vi "Drive Initialize.vi"(11 "Motor CAN IDs":T15={"Left Leader"=1, "Left Follower 1"=2, "Left Follower 2"=3, "Right Leader"=4, "Right Follower 1"=3, "Right Follower 2"=4}) -> (0 "Right Motor":T1={"DeviceStatus"={"status"=FALSE, "code"=0, "source"=""}, "Type"=enum."PWM", "PWM"={"PWM Channel"=enum."Invalid", "DeadBand"={"Name"="", "maxPositivePwm"=0, "minPositivePwm"=0, "centerPwm"=0, "maxNegativePwm"=0, "minNegativePwm"=0, "angularRange"=0}}, "CAN"={"Device Number"=0, "SetOutput VI Ref"=variant(refnum<vi> refnum), "GetOutput VI Ref"=variant(refnum<vi> refnum), "Enable VI Ref"=variant(refnum<vi> refnum), "Disable VI Ref"=variant(refnum<vi> refnum), "Data"=variant}, "Invert"=FALSE, "DIO PWM"={"PWM \"Enable\" Channel"=enum."Invalid", "DIOChannel"=enum."Invalid", "PWM Rate"=0.0}}, 1 "Left Motor":T1={"DeviceStatus"={"status"=FALSE, "code"=0, "source"=""}, "Type"=enum."PWM", "PWM"={"PWM Channel"=enum."Invalid", "DeadBand"={"Name"="", "maxPositivePwm"=0, "minPositivePwm"=0, "centerPwm"=0, "maxNegativePwm"=0, "minNegativePwm"=0, "angularRange"=0}}, "CAN"={"Device Number"=0, "SetOutput VI Ref"=variant(refnum<vi> refnum), "GetOutput VI Ref"=variant(refnum<vi> refnum), "Enable VI Ref"=variant(refnum<vi> refnum), "Disable VI Ref"=variant(refnum<vi> refnum), "Data"=variant}, "Invert"=FALSE, "DIO PWM"={"PWM \"Enable\" Channel"=enum."Invalid", "DIOChannel"=enum."Invalid", "PWM Rate"=0.0}}, 2 "imu":T6={"DevStatus"={"status"=FALSE, "code"=0, "source"=""}, "Hardware Config"={"SPI Clock Rate (Hz)"=1000000.0, "IMU SPI Mode (3)"=enum."Mode 3 (Clk Idle High,Sample on Trailing)", "IMU Reset Pin"=enum."SPI Port CS2", "IMU SPI Bus"=enum."SPI On-Board, CS0", "IMU Data Ready Pin"=enum."SPI Port CS1", "Stall Config"={"Pow2BytesPerRead"=255, "StallTicks"=640, "CsToSclkTicks"=5}, "IMU Status LED Pin"=enum."DIO MXP 9"}, "Calibration Complete"=refnum, "Status FIFO"=refnum, "Last Value Reference"=refnum, "Sychronous Process VI"=refnum, "Cmd FIFO"=refnum, "Source"={"DevStatus"={"status"=FALSE, "code"=0, "source"=""}, "AnalogTriggerMode?"=FALSE, "DigitalMode"={"DIO Channel"=enum."Disabled"}, "AnalogTriggerMode"={"AnalogTriggerIndex"=enum."Trig 0", "OutputType"=enum."InWindow"}}, "Data FIFO"=refnum, "IMU Status LED Pin"=enum."DIO MXP 9", "Calibration Time"=0}, 3 "Drive":T16)   [LabVIEW 2019]
uses:
  <vilib>/Rock Robotics/WPI/RobotDrive/WPI_RobotDriveDevRef.ctl
  <vilib>/Rock Robotics/WPI/MotorControl/WPI_MotorControlDeviceRef.ctl
  <vilib>/Rock Robotics/WPI/MotorControl/WPI_MotorControlType.ctl
  <vilib>/Rock Robotics/SystemInterfaces/DIO/FPGA_DIOPWMChannel.ctl
  <vilib>/Rock Robotics/WPI/PWM/WPI_PWMDeadband.ctl
  <vilib>/Rock Robotics/SystemInterfaces/DIO/FPGA_DIOChannel.ctl
  <vilib>/Rock Robotics/WPI/ThirdParty/ADI/ADIS16448/Typedef/ADIS16448 Device Reference.ctl
  <vilib>/Rock Robotics/WPI/ThirdParty/ADI/ADIS16448/Typedef/ADIS16448 Hardware Configuration.ctl
  <vilib>/Rock Robotics/WPI/SPI/WPI_SPIMode.ctl
  <vilib>/Rock Robotics/SystemInterfaces/spilib/spi_bus.ctl
  <vilib>/Rock Robotics/WPI/ThirdParty/ADI/ADIS16448/Typedef/ADIS16448 Status.ctl
  <vilib>/Rock Robotics/WPI/ThirdParty/ADI/ADIS16448/Typedef/ADIS16448 Data.ctl
  <vilib>/Rock Robotics/WPI/ThirdParty/ADI/ADIS16448/Typedef/ADIS16448 Process.ctl
  <vilib>/Rock Robotics/WPI/ThirdParty/ADI/ADIS16448/Typedef/ADIS16448 Command Type.ctl
  <vilib>/Rock Robotics/SystemInterfaces/CounterEncoderSourceConvertion/FPGA_CounterEncoderSourceConvertionLVSourceType.ctl
  <vilib>/Rock Robotics/SystemInterfaces/DIO/FPGA_DIODigitalSourceChannel.ctl
  <vilib>/Rock Robotics/SystemInterfaces/AnalogTrigger/FPGA_AnalogTriggerIndex.ctl
  <vilib>/Rock Robotics/SystemInterfaces/AnalogTrigger/FPGA_AnalogTriggerOutType.ctl
  <vilib>/Rock Robotics/WPI/SafetyOutput/WPI_SafetyOutputConfigMenu.ctl
  <vilib>/Rock Robotics/WPI/ThirdParty/REV Robotics/SPARK MAX/Typedef/Spark MAX Motor Type.ctl
  <vilib>/Rock Robotics/WPI/RobotDrive/WPI_RobotDriveOpen2MotorWithExistingMotors.vi
  Drive Published Globals.vi
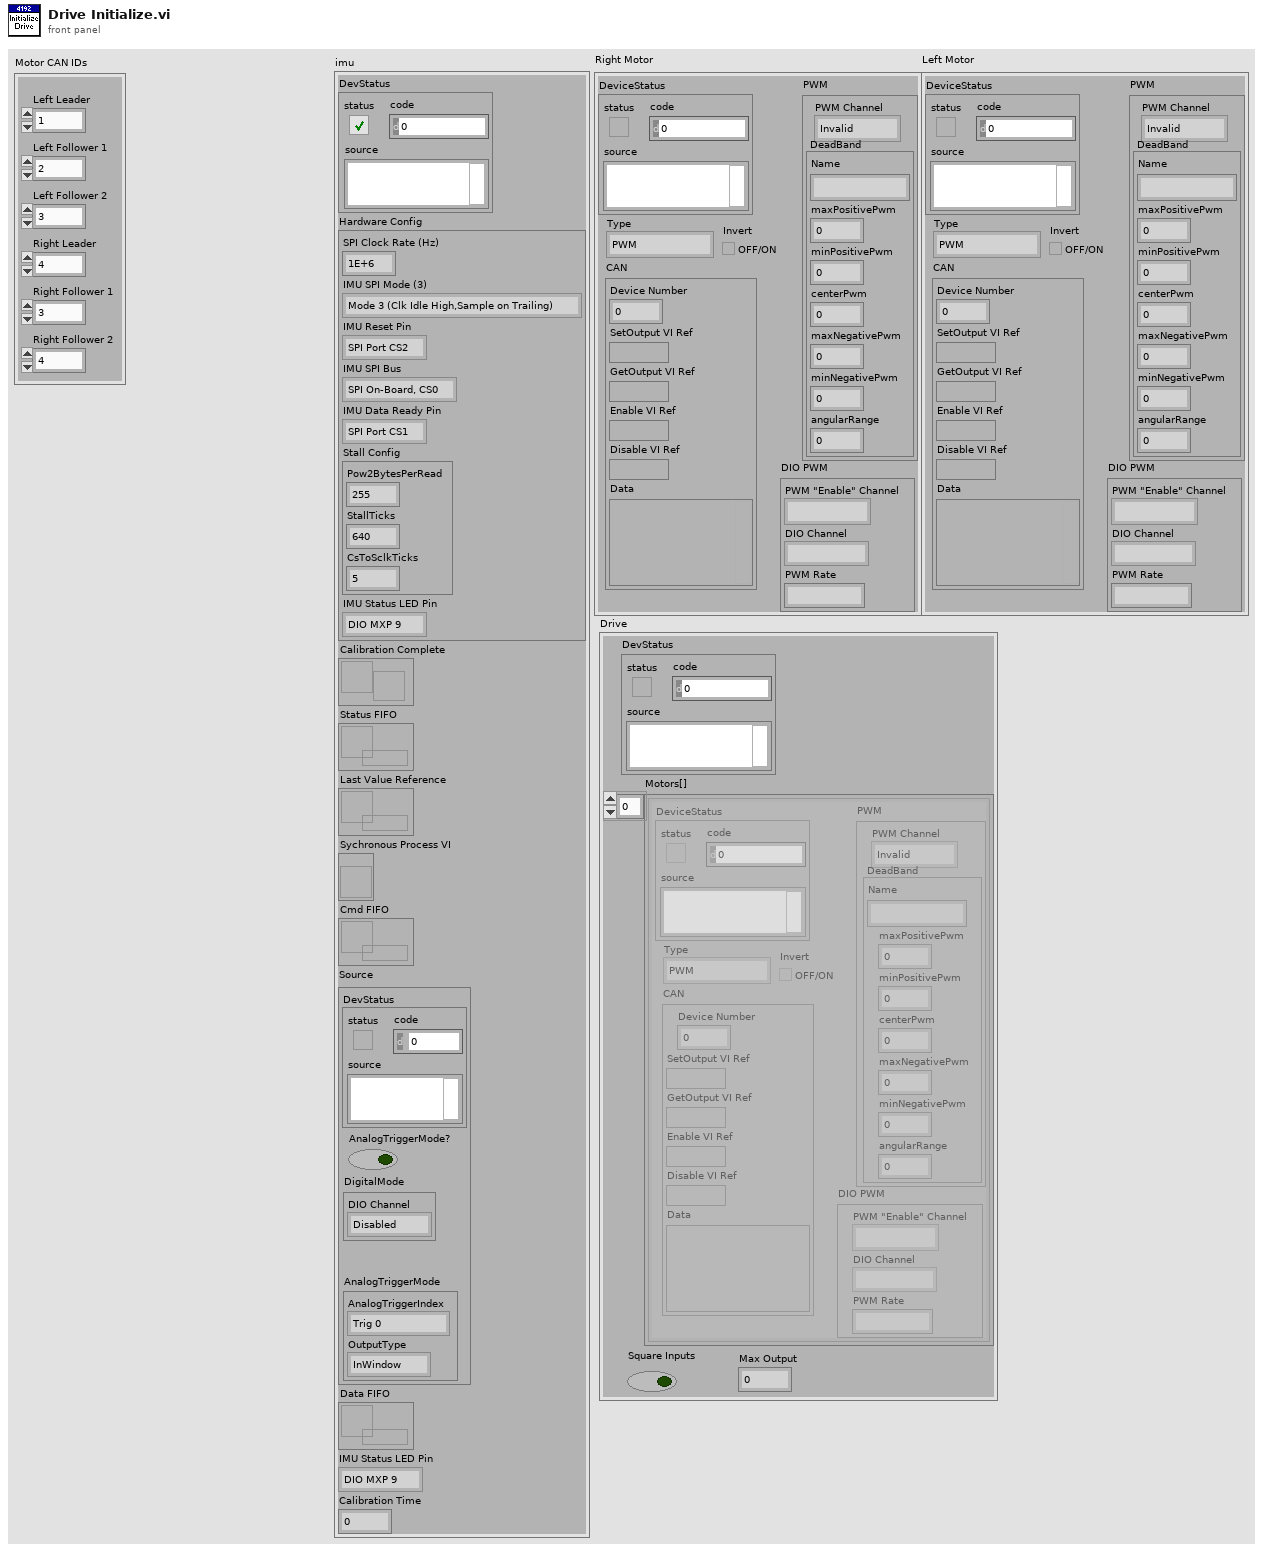
[diagram p1: front panel]
types:
  T1 = typedef "WPI_MotorControlDeviceRef.ctl" = cluster{"DeviceStatus":errorcluster, "Type":T2, "PWM":cluster{"PWM Channel":T3, "DeadBand":T4}, "CAN":cluster{"Device Number":u8, "SetOutput VI Ref":variant, "GetOutput VI Ref":variant, "Enable VI Ref":variant, "Disable VI Ref":variant, "Data":variant}, "Invert":bool, "DIO PWM":cluster{"PWM \"Enable\" Channel":T3, "DIOChannel":T5, "PWM Rate":dbl}}
  T2 = typedef "WPI_MotorControlType.ctl" = enum16{"PWM", "CAN", "DIO PWM"}
  T3 = typedef "FPGA_DIOPWMChannel.ctl" = enum8{"PWM 0", "PWM 1", "PWM 2", "PWM 3", "PWM 4", "PWM 5", "PWM 6", "PWM 7", "PWM 8", "PWM 9", "PWM MXP 0", "PWM MXP 1", "PWM MXP 2", "PWM MXP 3", "PWM MXP 4", "PWM MXP 5", "PWM MXP 6", "PWM MXP 7", "PWM MXP 8", "PWM MXP 9", "Invalid"}
  T4 = typedef "WPI_PWMDeadband.ctl" = cluster{"Name":string, "maxPositivePwm":i32, "minPositivePwm":i32, "centerPwm":i32, "maxNegativePwm":i32, "minNegativePwm":i32, "angularRange":u16}
  T5 = typedef "FPGA_DIOChannel.ctl" = enum8{"DIO 0", "DIO 1", "DIO 2", "DIO 3", "DIO 4", "DIO 5", "DIO 6", "DIO 7", "DIO 8", "DIO 9", "DIO MXP 0", "DIO MXP 1", "DIO MXP 2", "DIO MXP 3", "DIO MXP 4", "DIO MXP 5", "DIO MXP 6", "DIO MXP 7", "DIO MXP 8", "DIO MXP 9", "DIO MXP 10", "DIO MXP 11", "DIO MXP 12", "DIO MXP 13", "DIO MXP 14", "DIO MXP 15", "SPI Port CS1", "SPI Port CS2", "SPI Port CS3", "SPI Port MISO", "SPI Port MOSI", "Invalid"}
  T6 = typedef "ADIS16448 Device Reference.ctl" = cluster{"DevStatus":errorcluster, "Hardware Config":T7, "Calibration Complete":refnum<notifier>, "Status FIFO":refnum<k33>, "Last Value Reference":refnum<data-value>, "Sychronous Process VI":T10, "Cmd FIFO":refnum<k33>, "Source":T11, "Data FIFO":refnum<k33>, "IMU Status LED Pin":T5, "Calibration Time":u32}
  T7 = typedef "ADIS16448 Hardware Configuration.ctl" = cluster{"SPI Clock Rate (Hz)":dbl, "IMU SPI Mode (3)":T8, "IMU Reset Pin":T5, "IMU SPI Bus":T9, "IMU Data Ready Pin":T5, "Stall Config":cluster{"Pow2BytesPerRead":u8, "StallTicks":u16, "CsToSclkTicks":u8}, "IMU Status LED Pin":T5}
  T8 = typedef "WPI_SPIMode.ctl" = enum16{"Mode 0 (Clk Idle Low,Sample on Leading)", "Mode 1 (Clk Idle Low,Sample on Trailing)", "Mode 2 (Clk Idle High,Sample on Leading)", "Mode 3 (Clk Idle High,Sample on Trailing)"}
  T9 = typedef "spi_bus.ctl" = enum16{"SPI On-Board, CS0", "SPI On-Board, CS1", "SPI On-Board, CS2", "SPI On-Board, CS3", "SPI MXP", "Invalid"}
  T10 = typedef "ADIS16448 Process.ctl" = refnum<vi>
  T11 = typedef "FPGA_CounterEncoderSourceConvertionLVSourceType.ctl" = cluster{"DevStatus":errorcluster, "AnalogTriggerMode?":bool, "DigitalMode":cluster{"DIO Channel":T12}, "AnalogTriggerMode":cluster{"AnalogTriggerIndex":T13, "OutputType":T14}}
  T12 = typedef "FPGA_DIODigitalSourceChannel.ctl" = enum8{"DIO 0", "DIO 1", "DIO 2", "DIO 3", "DIO 4", "DIO 5", "DIO 6", "DIO 7", "DIO 8", "DIO 9", "DIO MXP 0", "DIO MXP 1", "DIO MXP 2", "DIO MXP 3", "DIO MXP 4", "DIO MXP 5", "DIO MXP 6", "DIO MXP 7", "DIO MXP 8", "DIO MXP 9", "DIO MXP 10", "DIO MXP 11", "DIO MXP 12", "DIO MXP 13", "DIO MXP 14", "DIO MXP 15", "SPI Port CS1", "SPI Port CS2", "SPI Port CS3", "SPI Port MISO", "SPI Port MOSI", "Disabled"}
  T13 = typedef "FPGA_AnalogTriggerIndex.ctl" = enum8{"Trig 0", "Trig 1", "Trig 2", "Trig 3", "Trig 4", "Trig 5", "Trig 6", "Trig 7", "Invalid"}
  T14 = typedef "FPGA_AnalogTriggerOutType.ctl" = enum16{"InWindow", "TriggerState", "Rising", "Falling"}
  T15 = cluster{"Left Leader":u8, "Left Follower 1":u8, "Left Follower 2":u8, "Right Leader":u8, "Right Follower 1":u8, "Right Follower 2":u8}
  T16 = typedef "WPI_RobotDriveDevRef.ctl" = cluster{"DevStatus":errorcluster, "Motors[]":T1[], "Square Inputs":bool, "Max Output":dbl}
  T17 = typedef "Spark MAX Motor Type.ctl" = enum16{"Brushed", "Brushless"}
  T18 = typedef "WPI_SafetyOutputConfigMenu.ctl" = enum16{"Enable", "Disable"}
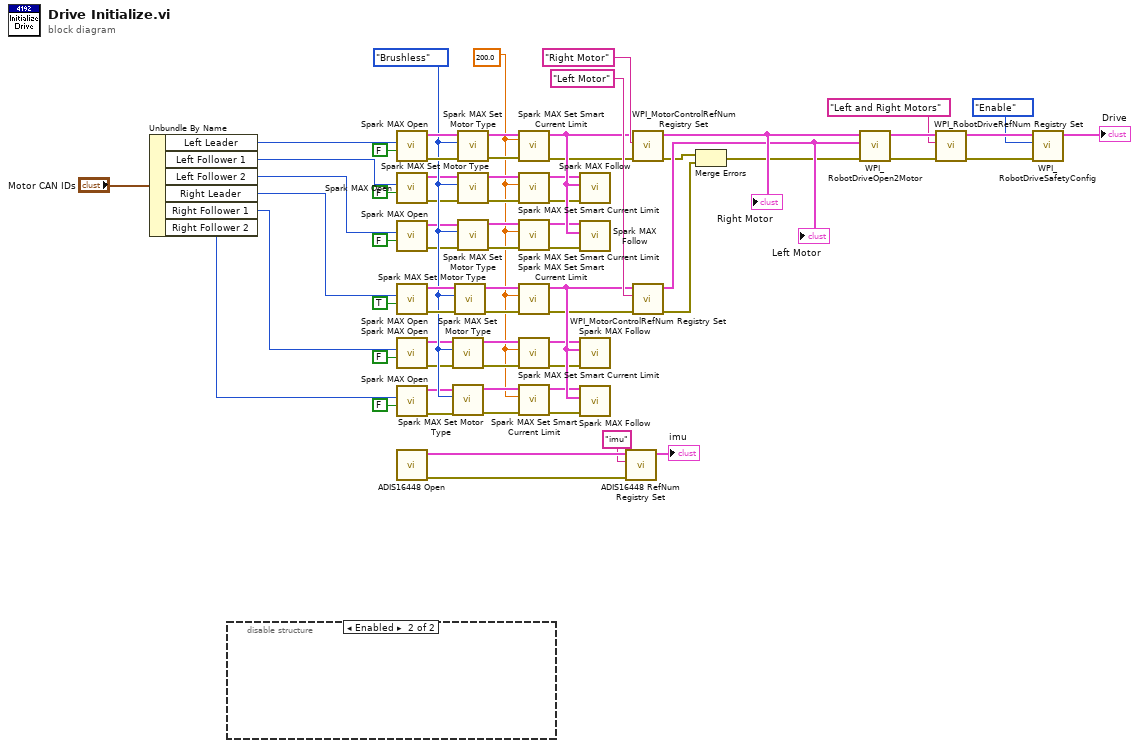
[diagram p0: block diagram]
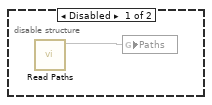
[diagram p2: hidden frame]
diagram:
  w7 = sgl 200.0 ("Current Limit A (100)")
  w61 = Spark_MAX_Motor_Type."Brushless" ("Motor Type")
  n1 = Unbundle By Name("Motor CAN IDs") -> ("Left Leader"=w57:u8, "Left Follower 1"=w32:u8, "Left Follower 2"=w60:u8, "Right Leader"=w59:u8, "Right Follower 1"=w58:u8, "Right Follower 2"=w39:u8)
  n2 = disable-structure shown="Enabled" {
    frame Disabled {
      n3 = call "Read Paths.vi"() -> ("Paths"=w70:map{string, dbl[][]})  [unwired: 11 in]
      n4 = global write "Drive Published Globals.vi" "Paths"(w70) -> ()
    }
    frame Enabled {
    }
  }
  n5 = call <vilib>:"Spark MAX Open.vi"("Invert"=FALSE, "Device Number"=w57) -> ("error out"=w67:errorcluster, "MotorControlDeviceRef"=w66:T1)  [unwired: 8 in]
  n6 = call <vilib>:"Spark MAX Open.vi"("Invert"=FALSE, "Device Number"=w32) -> ("error out"=w49:errorcluster, "MotorControlDeviceRef"=w50:T1)  [unwired: 8 in]
  n7 = call <vilib>:"Spark MAX Open.vi"("Invert"=FALSE, "Device Number"=w60) -> ("error out"=w47:errorcluster, "MotorControlDeviceRef"=w48:T1)  [unwired: 8 in]
  n8 = call <vilib>:"Spark MAX Open.vi"("Invert"=TRUE, "Device Number"=w59) -> ("error out"=w68:errorcluster, "MotorControlDeviceRef"=w69:T1)  [unwired: 8 in]
  n9 = call <vilib>:"Spark MAX Open.vi"("Invert"=FALSE, "Device Number"=w58) -> ("error out"=w53:errorcluster, "MotorControlDeviceRef"=w54:T1)  [unwired: 8 in]
  n10 = call <vilib>:"Spark MAX Open.vi"("Invert"=FALSE, "Device Number"=w39) -> ("error out"=w52:errorcluster, "MotorControlDeviceRef"=w51:T1)  [unwired: 8 in]
  n11 = call <vilib>:"ADIS16448 Open.vi"() -> ("error out"=w35:errorcluster, "ADIS16448DevRef"=w36:T6)  [unwired: 10 in]
  n12 = call <vilib>:"Spark MAX Set Motor Type.vi"("error in (no error)"=w53, "Motor Type"=w61, "MotorControlDevRef"=w54) -> ("error out"=w16:errorcluster, "MotorControlDeviceRef"=w17:T1)  [unwired: 7 in]
  n13 = call <vilib>:"Spark MAX Set Motor Type.vi"("error in (no error)"=w52, "Motor Type"=w61, "MotorControlDevRef"=w51) -> ("error out"=w14:errorcluster, "MotorControlDeviceRef"=w15:T1)  [unwired: 7 in]
  n14 = call <vilib>:"Spark MAX Set Motor Type.vi"("error in (no error)"=w68, "Motor Type"=w61, "MotorControlDevRef"=w69) -> ("error out"=w18:errorcluster, "MotorControlDeviceRef"=w19:T1)  [unwired: 7 in]
  n15 = call <vilib>:"Spark MAX Set Motor Type.vi"("error in (no error)"=w67, "Motor Type"=w61, "MotorControlDevRef"=w66) -> ("error out"=w30:errorcluster, "MotorControlDeviceRef"=w31:T1)  [unwired: 7 in]
  n16 = call <vilib>:"Spark MAX Set Motor Type.vi"("error in (no error)"=w49, "Motor Type"=w61, "MotorControlDevRef"=w50) -> ("error out"=w26:errorcluster, "MotorControlDeviceRef"=w27:T1)  [unwired: 7 in]
  n17 = call <vilib>:"Spark MAX Set Motor Type.vi"("error in (no error)"=w47, "Motor Type"=w61, "MotorControlDevRef"=w48) -> ("error out"=w22:errorcluster, "MotorControlDeviceRef"=w23:T1)  [unwired: 7 in]
  n18 = call <vilib>:"Spark MAX Set Smart Current Limit.vi"("error in (no error)"=w30, "Primay Current Limit (80A)"=w7, "MotorControlDeviceRef in"=w31) -> ("error out"=w28:errorcluster, "MotorControlDeviceRef out"=w29:T1)  [unwired: 7 in]
  n19 = call <vilib>:"Spark MAX Set Smart Current Limit.vi"("error in (no error)"=w26, "Primay Current Limit (80A)"=w7, "MotorControlDeviceRef in"=w27) -> ("error out"=w24:errorcluster, "MotorControlDeviceRef out"=w25:T1)  [unwired: 7 in]
  n20 = call <vilib>:"Spark MAX Set Smart Current Limit.vi"("error in (no error)"=w22, "Primay Current Limit (80A)"=w7, "MotorControlDeviceRef in"=w23) -> ("error out"=w20:errorcluster, "MotorControlDeviceRef out"=w21:T1)  [unwired: 7 in]
  n21 = call <vilib>:"Spark MAX Set Smart Current Limit.vi"("error in (no error)"=w18, "Primay Current Limit (80A)"=w7, "MotorControlDeviceRef in"=w19) -> ("error out"=w12:errorcluster, "MotorControlDeviceRef out"=w13:T1)  [unwired: 7 in]
  n22 = call <vilib>:"Spark MAX Set Smart Current Limit.vi"("error in (no error)"=w16, "Primay Current Limit (80A)"=w7, "MotorControlDeviceRef in"=w17) -> ("error out"=w10:errorcluster, "MotorControlDeviceRef out"=w11:T1)  [unwired: 7 in]
  n23 = call <vilib>:"Spark MAX Set Smart Current Limit.vi"("error in (no error)"=w14, "Primay Current Limit (80A)"=w7, "MotorControlDeviceRef in"=w15) -> ("error out"=w8:errorcluster, "MotorControlDeviceRef out"=w9:T1)  [unwired: 7 in]
  n24 = call <vilib>:"Spark MAX Follow.vi"("error in (no error)"=w24, "Master Controller"=w29, "MotorControlDeviceRef"=w25) -> ()  [unwired: 7 in, 2 out]
  n25 = call <vilib>:"Spark MAX Follow.vi"("error in (no error)"=w20, "Master Controller"=w29, "MotorControlDeviceRef"=w21) -> ()  [unwired: 7 in, 2 out]
  n26 = call <vilib>:"Spark MAX Follow.vi"("error in (no error)"=w10, "Master Controller"=w13, "MotorControlDeviceRef"=w11) -> ()  [unwired: 7 in, 2 out]
  n27 = call <vilib>:"Spark MAX Follow.vi"("error in (no error)"=w8, "Master Controller"=w13, "MotorControlDeviceRef"=w9) -> ()  [unwired: 7 in, 2 out]
  n28 = call <vilib>:"ADIS16448 RefNum Registry Set.vi"("error in (no error)"=w35, "refnum name"="imu", "ADIS16448DevRef"=w36) -> ("ADIS16448DevRef Out"=→"imu":T6)  [unwired: 7 in, 1 out]
  n29 = call <vilib>:"WPI_MotorControlRefNum Registry Set.vi"("error in (no error)"=w28, "refnum name"="Right Motor", "MotorControlDevRef"=w29) -> ("error out"=w56:errorcluster, "MotorControlDevRef"=w65:T1)  [unwired: 7 in]
  "Right Motor" <- w65
  n30 = call <vilib>:"WPI_MotorControlRefNum Registry Set.vi"("error in (no error)"=w12, "refnum name"="Left Motor", "MotorControlDevRef"=w13) -> ("error out"=w55:errorcluster, "MotorControlDevRef"=w63:T1)  [unwired: 7 in]
  "Left Motor" <- w63
  n31 = Merge Errors(w56, w55) -> (w46:errorcluster)
  n32 = call-poly <vilib>:"WPI_RobotDriveOpen2Motor.vi"("error in (no error)"=w46, "Right Motor Dev Ref"=w63, "Left Motor Dev Ref"=w65) -> ("error out"=w44:errorcluster, "RobotDriveDevRef"=w45:T16)  [unwired: 7 in]
  n33 = call <vilib>:"WPI_RobotDriveRefNum Registry Set.vi"("error in (no error)"=w44, "refnum name"="Left and Right Motors", "RobotDriveDevRef"=w45) -> ("error out"=w43:errorcluster, "RobotDriveDevRef"=w42:T16)  [unwired: 1 in, 6 out]
  n34 = call <vilib>:"WPI_RobotDriveSafetyConfig.vi"("error in (no error)"=w43, "mode"=WPI_SafetyOutputConfigMenu."Enable", "RobotDriveDevRef"=w42) -> ("RobotDriveDevRef"=→"Drive":T16)  [unwired: 7 in, 1 out]
